vi "Get 8 Neighbors.vi"(9 "column":i32, 10 "row":i32, 11 "cells in":bool[][](array[boolean])) -> (3 "cells living":bool[](array[boolean]))   [LabVIEW 2024, in "Game Of Life.lvlib"]
uses:
  Game Of Life.lvlib
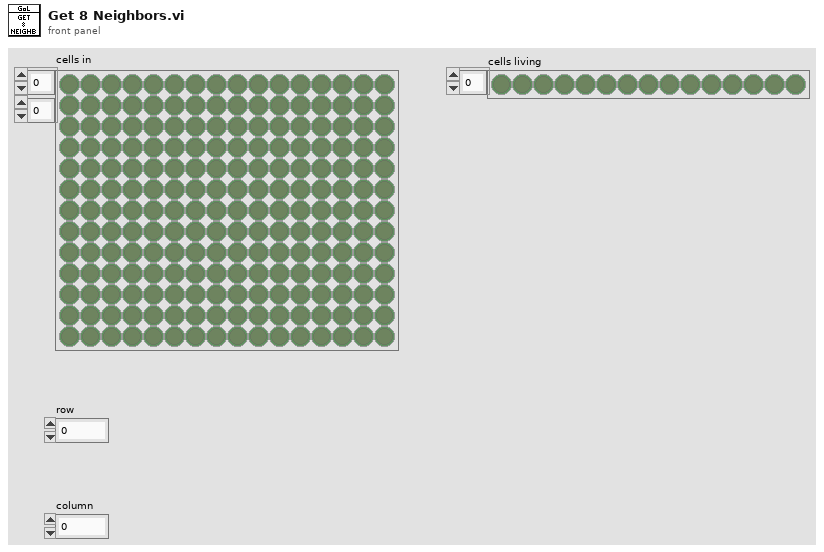
[diagram p1: front panel]
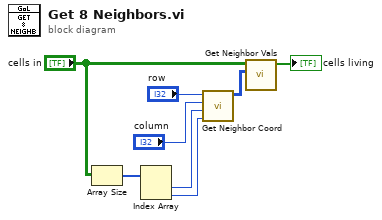
[diagram p0: block diagram]
diagram:
  n1 = Array Size(array="cells in") -> (size(s)=w8:i32[])
  n2 = Index Array(array=w8) -> (element #1=w5:i32, element #2=w4:i32)  [unwired: 2 in]
  n3 = call "Get Neighbor Coord.vi"("# cols"=w4, "# rows"=w5, "column"="column", "row"="row") -> ("neighbor coordinates"=w2:i32[][])  [unwired: 7 in]
  n4 = call "Get Neighbor Vals.vi"("neighbor coordinates"=w2, "cells in"="cells in") -> ("cells living"=→"cells living":bool[])  [unwired: 9 in]
